vi "Test Pass if Equal 1el String Arrays.vi"(8 "error in (no error)":errorcluster, 11 "Compare Assertion Test In":refnum<class "Compare Assertion Test.lvclass">) -> (0 "error out":errorcluster, 3 "Compare Assertion Test Out":refnum<class "Compare Assertion Test.lvclass">)   [LabVIEW 2020, in "Compare Assertion Test.lvclass"]
uses:
  Compare Assertion Test.lvclass
  C:/Program Files (x86)/National Instruments/LabVIEW 2020/vi.lib/Astemes/LUnit/Test Case.lvclass
  Comparison Test Double/Test Methods.ctl
  <vilib>/Astemes/LUnit/Test Case.lvclass/Test Case.ctl
  986b99f8-79ab-40b1-b6ba-050484e839cd.vi
  <vilib>/Astemes/LUnit/Append Pass Result.vi
  <vilib>/Astemes/LUnit/Append Fail Result.vi
  <vilib>/Astemes/LUnit/Describe Comparison.vi
  986b99f8-79ab-40b1-b6ba-050484e839cd.vi/9c5d11cd-9439-4240-a1ee-d9baace9c924.vi
  <vilib>/Astemes/LUnit/Run In UI.vi
  <vilib>/Utility/error.llb/Clear Errors.vi
  <vilib>/Astemes/LUnit/Describe Variant.vi
  Comparison Test Double/Comparison Test Double.lvclass
panel:
  out "error out 2":errorcluster
  out "Message":string
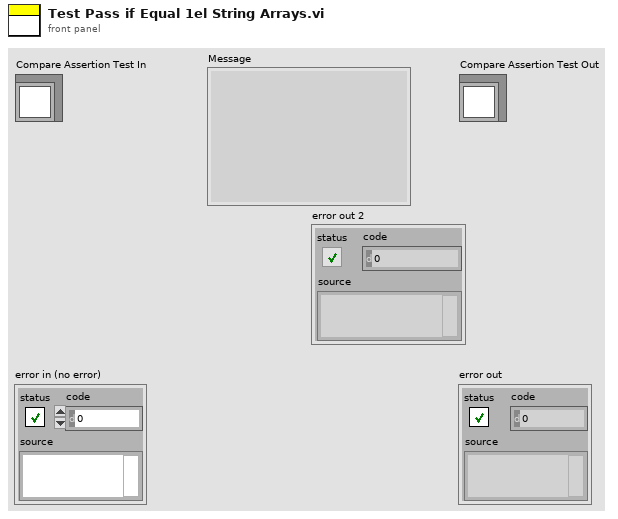
[diagram p1: front panel]
types:
  T1 = typedef "Comparison Test Double.lvclass/Test Methods.ctl" = enum16{"Test Compare Equal Enums.vi", "Test Compare Unequal Enums.vi", "Test Compare Equal Strings.vi", "Test Compare Unequal Type Deffed Enums.vi", "Test Compare Equal 8bit Enums.vi", "Test Compare Equal 1el String Arrays.vi", "Test Compare Fail if Equal 1el String Arrays.vi", "Test Compare Array with Tolerance.vi", "Test Compare Equal Strings one as Variant.vi", "Test Compare Equal Strings Other as Variant.vi", "Test Compare Equal Variants.vi"}
  T2 = typedef "Result.lvlib/Result.ctl" = cluster{"Name":string, "Message":string, "Description":string, "Status":T3, "Result Type":T4, "Execution Time":dbl}
  T3 = typedef "Result.lvlib/Status.ctl" = enum16{"", "Passed", "Failed", "Error", "Skipped", "Setup Error", "Broken", "Teardown Error"}
  T4 = typedef "Result.lvlib/Type.ctl" = enum16{"Test Case", "Test Suite", "Test Run", "Pass", "Fail", "Skip", "Pass if", "Fail if", "Pass if Error", "Fail if Error", "Pass if Equal", "Fail if Equal"}
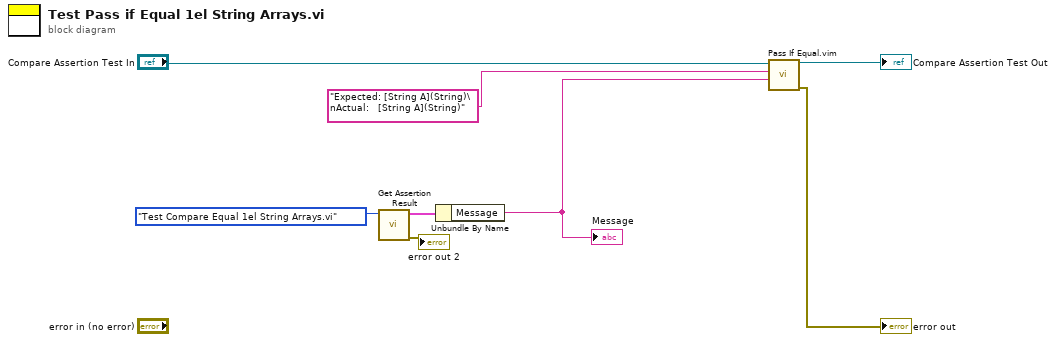
[diagram p0: block diagram]
diagram:
  n1 = call "Get Assertion Result.vi"("Test VIs"=Test_Methods."Test Compare Equal 1el String Arrays.vi") -> ("error out"=→"error out 2":errorcluster, "First Result"=w5:T2)  [unwired: 8 in, 1 out]
  n2 = Unbundle By Name(w5) -> ("Message"=w4:string)
  "Message" <- w4
  n3 = call "Pass If Equal.vim"("Actual"=w4, "Expected"="Expected: [String A](String)\nActual:   [String A](String)" ("Message"), "LUnit Test Case In"="Compare Assertion Test In") -> ("error out"=→"error out":errorcluster, "LUnit Test Case Out"=→"Compare Assertion Test Out":refnum<class "Compare Assertion Test.lvclass">)  [unwired: 7 in]
